vi "Find Positive Transitions.vi"(11 "Boolean Array in":bool[](array[boolean])) -> (3 "Positive Transitions":bool[](array[boolean]))   [LabVIEW 2018, in "Image Management.lvlib"]
uses:
  Image Management.lvlib
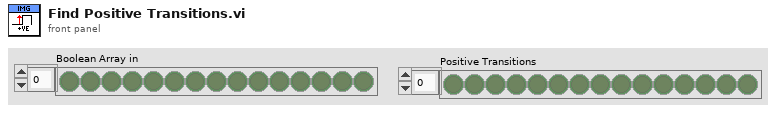
[diagram p1: front panel]
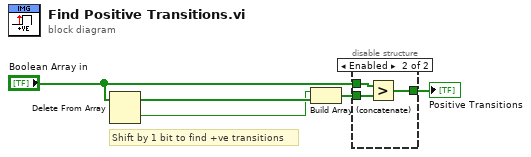
[diagram p0: block diagram]
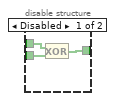
[diagram p2: hidden frame]
diagram:
  # "Shift by 1 bit to find +ve transitions"
  n1 = Delete From Array(array="Boolean Array in") -> (deleted portion=w1:bool, array with subset deleted=w2:bool[])  [unwired: 2 in]
  n2 = Build Array (concatenate)(w1, w2) -> (w3:bool[])
  n3 = disable-structure shown="Enabled" {
    disable-tunnel: w3 -> [w8 w10]
    disable-tunnel: [w7 w9] -> w5
    disable-tunnel: "Boolean Array in" -> [w6 w11]
    frame Disabled {
      n4 = Exclusive Or(1:w8, 2:w6) -> (0:w7:bool[])
    }
    frame Enabled {
      n5 = Greater?(x=w11, y=w10) -> (0:w9:bool[])
    }
  }
  "Positive Transitions" <- w5
